vi "outputTOcluster.vi"(7 "Input":string, 11 "error in (no error)":errorcluster) -> (8 "String":string, 10 "Set_lower":T2, 15 "error out":errorcluster)   [LabVIEW 2014, in "FH 55.lvlib"]
uses:
  FH 55.lvlib
  TypeDef/Unit2.ctl
panel:
  in  "Set_lower 2":T2
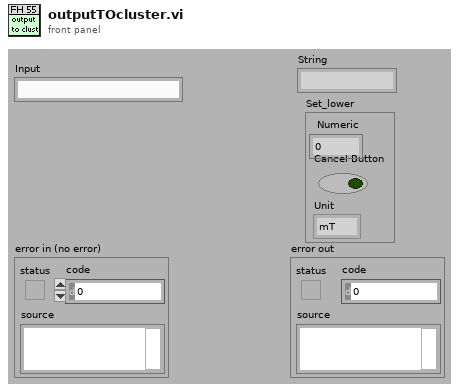
[diagram p1: front panel]
types:
  T1 = typedef "FH 55.lvlib/Unit2.ctl" = enum16{"mT", "G", "kA/m"}
  T2 = cluster{"Numeric":dbl, "Cancel Button":bool, "Unit":T1}
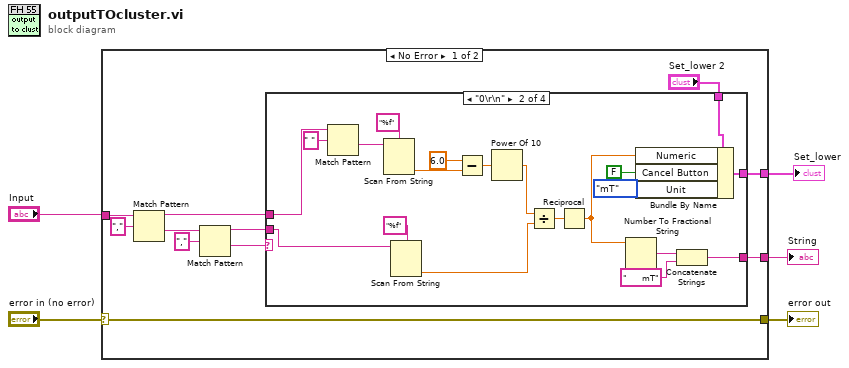
[diagram p0: block diagram]
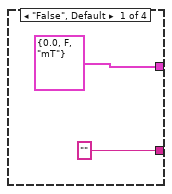
[diagram p2: hidden frame]
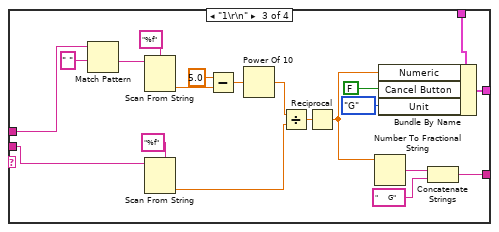
[diagram p3: hidden frame]
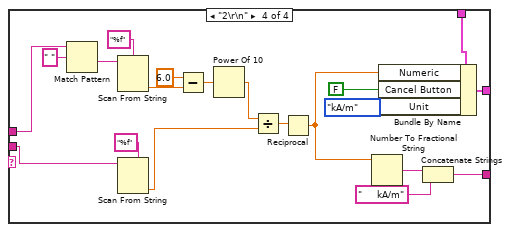
[diagram p4: hidden frame]
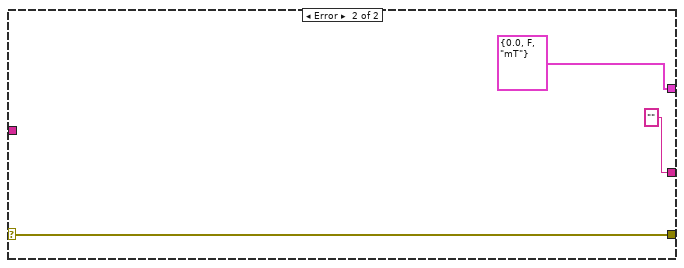
[diagram p5: hidden frame]
diagram:
  n1 = case shown="No Error" "error in (no error)" {
    selector: "error in (no error)" -> [w8 w81]
    tunnel: [w8 w81] -> w4
    tunnel: "Input" -> [w15 _]
    tunnel: [w9 ""] -> w2
    tunnel: [w6 T2 {"Numeric"=0.0, "Cancel Button"=FALSE, "Unit"=enum."mT"} ("Set_lower")] -> w1
    frame No Error {
      n2 = Match Pattern(string=w15, regular expression=",") -> (before substring=w10:string, after substring=w14:string)  [unwired: 1 in, 2 out]
      n3 = Match Pattern(string=w14, regular expression=",") -> (before substring=w12:string, after substring=w11:string)  [unwired: 1 in, 2 out]
      n4 = case shown="\"0\\r\\n\"" w11 {
        tunnel: w12 -> [_ w19 w39 w59]
        tunnel: w10 -> [_ w31 w51 w71]
        tunnel: ["" w26 w46 w66] -> w9
        tunnel: "Set_lower 2" -> [_ w21 w45 w63]
        tunnel: [T2 {"Numeric"=0.0, "Cancel Button"=FALSE, "Unit"=enum."mT"} ("Set_lower") w20 w40 w60] -> w6
        frame "False", Default {
        }
        frame "0\r\n" {
          n5 = Match Pattern(string=w31, regular expression=" ") -> (after substring=w32:string)  [unwired: 1 in, 3 out]
          n6 = Scan From String(format string="%f", input string=w32) -> (output 1=w35:dbl)  [unwired: 3 in, 3 out]
          n7 = Scan From String(format string="%f", input string=w19) -> (output 1=w25:dbl)  [unwired: 3 in, 3 out]
          n8 = Subtract(x=6.0, y=w35) -> (x-y=w34:dbl)
          n9 = Power Of 10(x=w34) -> (10^x=w24:dbl)
          n10 = Divide(x=w24, y=w25) -> (x/y=w23:dbl)
          n11 = Reciprocal(x=w23) -> (1/x=w22:dbl)
          n12 = Number To Fractional String(number=w22) -> (F-format string=w30:string)  [unwired: 3 in]
          n13 = Bundle By Name(cluster=w21, "Numeric"=w22, "Cancel Button"=FALSE, "Unit"=Unit2."mT") -> (w20:T2)
          n14 = Concatenate Strings(w30, "     mT" ("string")) -> (w26:string)
        }
        frame "1\r\n" {
          n15 = Match Pattern(string=w51, regular expression=" ") -> (after substring=w52:string)  [unwired: 1 in, 3 out]
          n16 = Scan From String(format string="%f", input string=w52) -> (output 1=w55:dbl)  [unwired: 3 in, 3 out]
          n17 = Scan From String(format string="%f", input string=w39) -> (output 1=w43:dbl)  [unwired: 3 in, 3 out]
          n18 = Subtract(x=5.0, y=w55) -> (x-y=w54:dbl)
          n19 = Power Of 10(x=w54) -> (10^x=w44:dbl)
          n20 = Divide(x=w44, y=w43) -> (x/y=w42:dbl)
          n21 = Reciprocal(x=w42) -> (1/x=w41:dbl)
          n22 = Number To Fractional String(number=w41) -> (F-format string=w50:string)  [unwired: 3 in]
          n23 = Bundle By Name(cluster=w45, "Numeric"=w41, "Cancel Button"=FALSE, "Unit"=Unit2."G") -> (w40:T2)
          n24 = Concatenate Strings(w50, "     G" ("string")) -> (w46:string)
        }
        frame "2\r\n" {
          n25 = Match Pattern(string=w71, regular expression=" ") -> (after substring=w72:string)  [unwired: 1 in, 3 out]
          n26 = Scan From String(format string="%f", input string=w72) -> (output 1=w75:dbl)  [unwired: 3 in, 3 out]
          n27 = Scan From String(format string="%f", input string=w59) -> (output 1=w64:dbl)  [unwired: 3 in, 3 out]
          n28 = Subtract(x=6.0, y=w75) -> (x-y=w74:dbl)
          n29 = Power Of 10(x=w74) -> (10^x=w65:dbl)
          n30 = Divide(x=w65, y=w64) -> (x/y=w62:dbl)
          n31 = Reciprocal(x=w62) -> (1/x=w61:dbl)
          n32 = Number To Fractional String(number=w61) -> (F-format string=w70:string)  [unwired: 3 in]
          n33 = Bundle By Name(cluster=w63, "Numeric"=w61, "Cancel Button"=FALSE, "Unit"=Unit2."kA/m") -> (w60:T2)
          n34 = Concatenate Strings(w70, "     kA/m" ("string")) -> (w66:string)
        }
      }
    }
    frame Error {
    }
  }
  "error out" <- w4
  "String" <- w2
  "Set_lower" <- w1
